vi "Test Boards_OO.vi"() -> ()   [LabVIEW 2018]
doc: "See <b>Read_Me.html</b> in the <b>Board Testing</b> project for a detailed description of this VI."
uses:
  Common/Board Image.ctl
  Classes/Assembly Line Input_class/Assembly Line Input.lvclass
  Classes/Board Design_class/Board Design.lvclass
panel:
  out "Test Results":T2(array[cluster])
  # "Overview: Demonstrates a task-based solution to a board testing problem.\n\nSee Read_Me.html in the project for a detailed description of this VI."
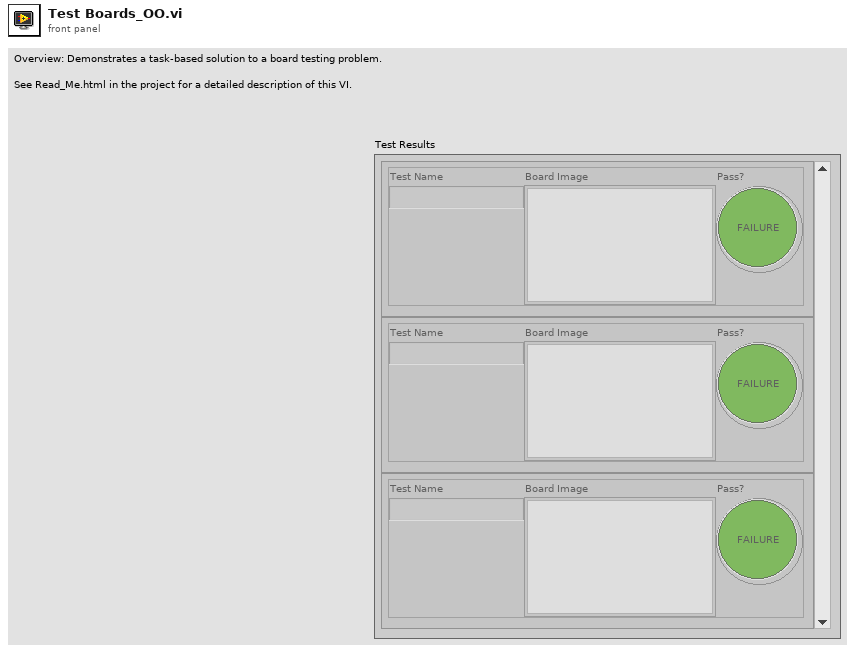
[diagram p1: front panel]
types:
  T1 = typedef "Board Image.ctl" = picture
  T2 = cluster{"Test Name":string, "Board Image":T1, "Pass?":bool}[]
  T3 = typedef "Board Type Enum.ctl" = enum16{"Basic DAQ Board", "Elite DAQ Board", "GPIB Board"}
  T4 = typedef "Pass Fail Boolean.ctl" = bool
  T5 = cluster{"Test name":string, "Accessors:board image":T1, "pass?":T4}
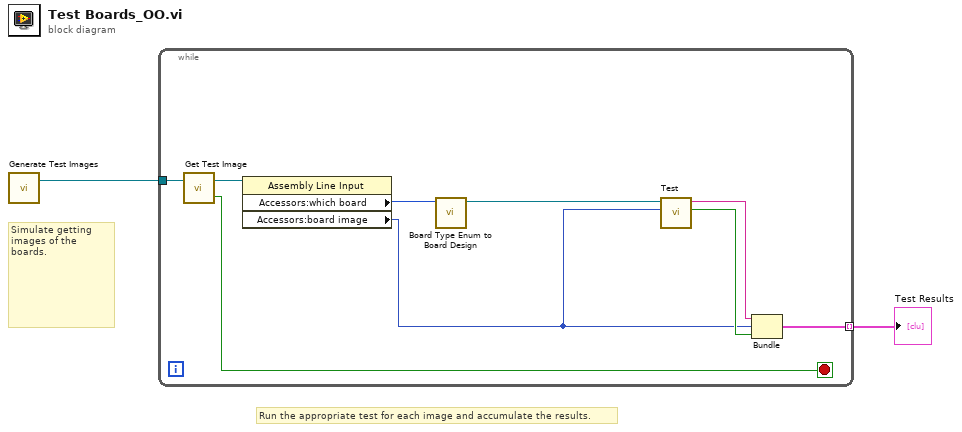
[diagram p0: block diagram]
diagram:
  # "Run the appropriate test for each image and accumulate the results."
  # "Simulate getting images of the boards."
  n1 = call "Generate Test Images.vi"() -> ("queue out"=w2:refnum<queue>)  [unwired: 2 in, 1 out]
  n2 = while {
    tunnel: w2 -> [w11]
    tunnel: [w9] -> w1 mode=indexing
    stop <- w10 stop-if-true
    n3 = call "Get Test Image.vi"("queue in"=w11) -> ("no more images after this?"=w10:bool, "Assembly Line Input"=w8:refnum<class "Assembly Line Input.lvclass">)  [unwired: 1 in]
    n4 = property class="Assembly Line Input"(reference=w8) -> ("Accessors:which board"=w7:T3, "Accessors:board image"=w3:T1)  [unwired: 1 in, 2 out]
    n5 = call "Board Type Enum to Board Design.vi"("which board"=w7) -> ("Board Design"=w6:refnum<class "Board Design.lvclass">)  [unwired: 10 in]
    n6 = call-dynamic "Test.vi"("board image"=w3, "Board Design in"=w6) -> ("pass?"=w4:T4, "Test name"=w5:string)  [unwired: 7 in, 1 out]
    n7 = Bundle("Test name"=w5, "Accessors:board image"=w3, "pass?"=w4) -> (w9:T5)  [unwired: 1 in]
  }
  "Test Results" <- w1
